vi "Configure Internal Control.vi"(8 "error in (no error)":errorcluster, 10 "Internal Control":bool, 11 "VISA resource name":refnum<visa-resource-name>) -> (0 "error out":errorcluster, 3 "VISA resource name out":refnum<visa-resource-name>)   [LabVIEW 2022 SP3, in "MagnaDC.lvlib"]
uses:
  MagnaDC.lvlib
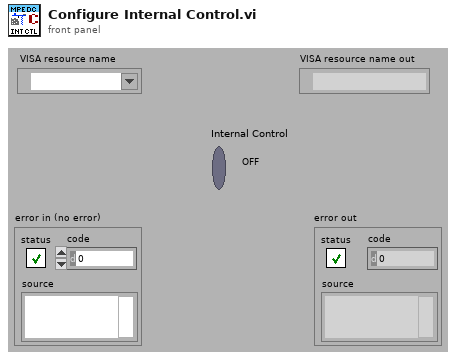
[diagram p1: front panel]
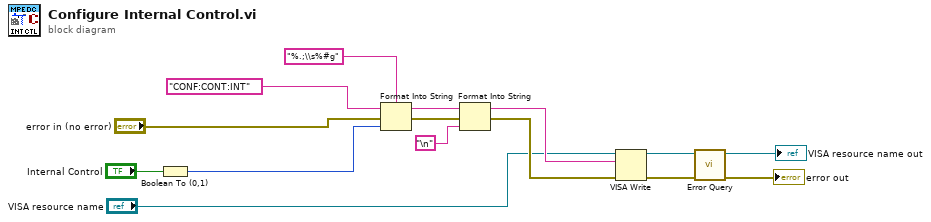
[diagram p0: block diagram]
diagram:
  n1 = Boolean To (0,1)(Boolean="Internal Control") -> (0, 1=w1:i16)
  n2 = Format Into String(format string="%.;\\s%#g", initial string="CONF:CONT:INT" ("format string"), error in="error in (no error)", w1) -> (resulting string=w3:string, error out=w4:errorcluster)
  n3 = Format Into String(initial string=w3, error in=w4, "\n") -> (resulting string=w9:string, error out=w11:errorcluster)  [unwired: 1 in]
  n4 = VISA Write(VISA resource name="VISA resource name", write buffer=w9, error in (no error)=w11) -> (VISA resource name out=w13:refnum<visa-resource-name>, error out=w12:errorcluster)  [unwired: 1 out]
  n5 = call "Error Query.vi"("error in (no error)"=w12, "VISA resource name"=w13) -> ("error out"=→"error out":errorcluster, "VISA resource name out"=→"VISA resource name out":refnum<visa-resource-name>)  [unwired: 6 in, 2 out]
